vi "Borda_Subida_Segurança.vi"(1 "Entrada":bool) -> (0 "Boolean":bool)   [LabVIEW 2018]
panel:
  in  "Aux Muda":bool
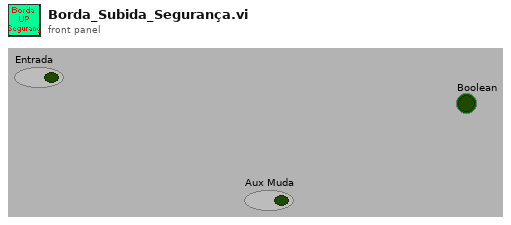
[diagram p1: front panel]
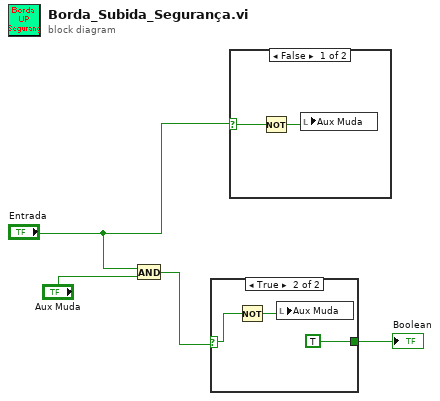
[diagram p0: block diagram]
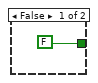
[diagram p3: hidden frame]
diagram:
  n1 = And(x="Entrada", y="Aux Muda") -> (x .and. y?=w2:bool)
  n2 = case shown="True" w2 {
    selector: w2 -> [_ w6]
    tunnel: [FALSE ("Boolean") TRUE ("Boolean")] -> w4
    frame False {
    }
    frame True {
      n3 = Not(x=w6) -> (.not. x?=w7:bool)
      n4 = local write "Aux Muda"(w7) -> ()
    }
  }
  "Boolean" <- w4
  n5 = case shown="False" "Entrada" {
    selector: "Entrada" -> [w10 _]
    frame False {
      n6 = Not(x=w10) -> (.not. x?=w9:bool)
      n7 = local write "Aux Muda"(w9) -> ()
    }
    frame True {
    }
  }
